vi "PM9_TCP_MODE.vi"(0 "VISA":refnum<visa-resource-name>="TCPIP0::169.254.70.190::502::SOCKET", 5 "connection ID":refnum<k5>, 11 "error in (no error)":errorcluster, 13 "MODE":u16(ring) items=["READ ONLY"=0, "AUTO"=10, "OFF"=62, "MAN"=54], 14 "Close tcp(t)":bool) -> (3 "mode(read)":string="OFF", 4 "visa out":refnum<visa-resource-name>, 6 "connection ID out":refnum<k5>, 15 "error out":errorcluster)   [LabVIEW 2018]
panel:
  # "Use a valid connection id to run in loop"
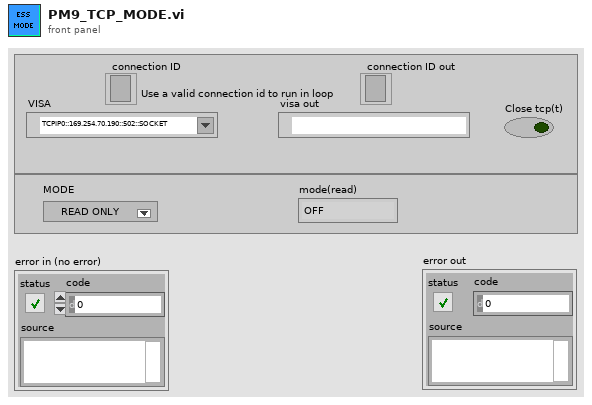
[diagram p1: front panel]
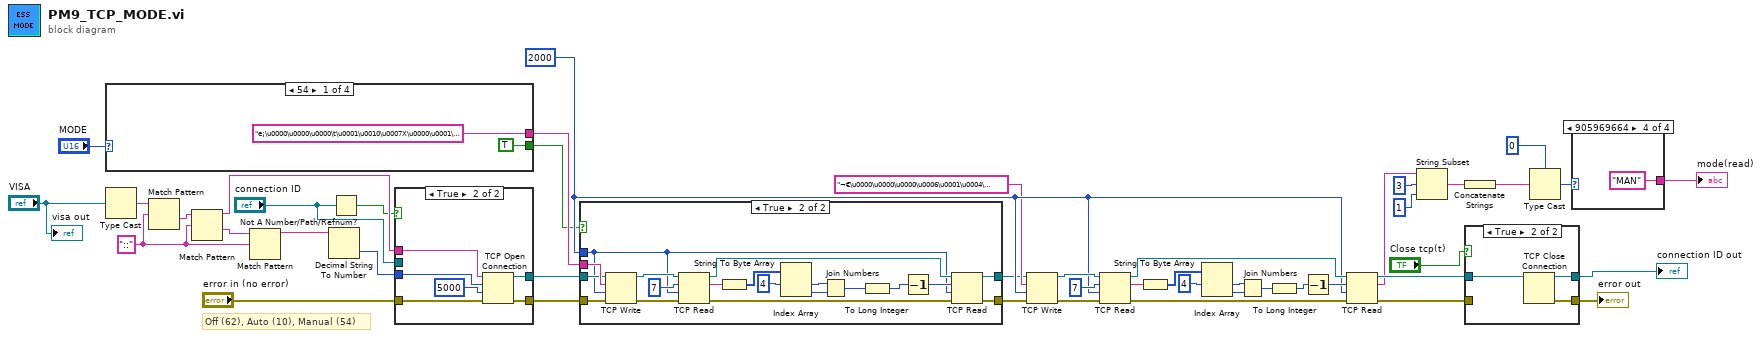
[diagram p0: block diagram]
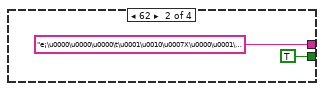
[diagram p3: hidden frame]
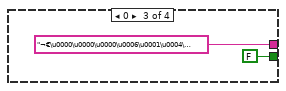
[diagram p4: hidden frame]
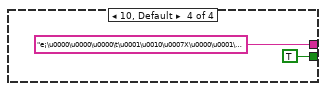
[diagram p5: hidden frame]
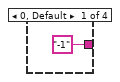
[diagram p6: hidden frame]
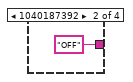
[diagram p7: hidden frame]
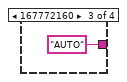
[diagram p8: hidden frame]
diagram:
  w38 = "::" ("search string/char (-)")
  w9 = 2000 ("timeout ms (25000)")
  # "Off (62), Auto (10), Manual (54)"
  n1 = case shown="54" "MODE" {
    tunnel: ["e¡\u0000\u0000\u0000\t\u0001\u0010\u0007X\u0000\u0001\u0002\u00006" ("address") "e¡\u0000\u0000\u0000\t\u0001\u0010\u0007X\u0000\u0001\u0002\u0000>" ("address") "¬€\u0000\u0000\u0000\u0006\u0001\u0004\u0007X\u0000\u0002" ("address") "e¡\u0000\u0000\u0000\t\u0001\u0010\u0007X\u0000\u0001\u0002\u0000\n" ("address")] -> w27
    tunnel: [TRUE TRUE FALSE TRUE] -> w5
    frame 54 {
    }
    frame 62 {
    }
    frame 0 {
    }
    frame 10, Default {
    }
  }
  n2 = Type Cast(x="VISA") -> (*(type *) &x=w41:string)  [unwired: 1 in]
  n3 = Match Pattern(string=w41, regular expression=w38) -> (after substring=w40:string)  [unwired: 1 in, 3 out]
  n4 = Match Pattern(string=w40, regular expression=w38) -> (before substring=w36:string, after substring=w39:string)  [unwired: 1 in, 2 out]
  n5 = Match Pattern(string=w39, regular expression=w38) -> (before substring=w37:string)  [unwired: 1 in, 3 out]
  n6 = Decimal String To Number(string=w37) -> (number=w35:i32)  [unwired: 2 in, 1 out]
  n7 = Not A Number/Path/Refnum?(number/path/refnum="connection ID") -> (NaN/Path/Refnum?=w30:bool)
  n8 = case shown="True" w30 {
    tunnel: [w56 w62] -> w4
    tunnel: [w55 w61] -> w46
    tunnel: w36 -> [_ w59]
    tunnel: w35 -> [_ w58]
    tunnel: "error in (no error)" -> [w55 w57]
    tunnel: "connection ID" -> [w56 _]
    frame False {
    }
    frame True {
      n9 = TCP Open Connection(address=w59, remote port or service name=w58, timeout ms (60000)=5000, error in (no error)=w57) -> (connection ID=w62:refnum<k5>, error out=w61:errorcluster)  [unwired: 1 in]
    }
  }
  n10 = case shown="True" w5 {
    tunnel: w46 -> [w64 w83]
    tunnel: w27 -> [_ w69]
    tunnel: w4 -> [w63 w68]
    tunnel: [w64 w67] -> w11
    tunnel: w9 -> [_ w66]
    tunnel: [w63 w65] -> w7
    frame False {
    }
    frame True {
      n11 = TCP Write(connection ID=w68, data in=w69, error in (no error)=w83, 9:w66) -> (connection ID out=w82:refnum<k5>, error out=w80:errorcluster)  [unwired: 1 out]
      n12 = TCP Read(connection ID=w82, bytes to read=7, error in (no error)=w80, 9:w66) -> (connection ID out=w81:refnum<k5>, data out=w71:string, error out=w79:errorcluster)  [unwired: 1 in]
      n13 = String To Byte Array(string=w71) -> (unsigned byte array=w72:u8[])
      n14 = Index Array(array=w72, index #1=4 ("index")) -> (element #1=w73:u8, element #2=w74:u8)  [unwired: 1 in]
      n15 = Join Numbers(hi=w73, lo=w74) -> ((hi.lo)=w76:u16)
      n16 = To Long Integer(number=w76) -> (32bit integer=w75:i32)
      n17 = Decrement(x=w75) -> (x-1=w70:i32)
      n18 = TCP Read(connection ID=w81, bytes to read=w70, error in (no error)=w79, 9:w66) -> (connection ID out=w65:refnum<k5>, error out=w67:errorcluster)  [unwired: 1 in, 1 out]
    }
  }
  n19 = TCP Write(connection ID=w7, data in="¬€\u0000\u0000\u0000\u0006\u0001\u0004\u0007X\u0000\u0002" ("address"), error in (no error)=w11, 9:w9) -> (connection ID out=w12:refnum<k5>, error out=w14:errorcluster)  [unwired: 1 out]
  n20 = TCP Read(connection ID=w12, bytes to read=7, error in (no error)=w14, 9:w9) -> (connection ID out=w13:refnum<k5>, data out=w23:string, error out=w15:errorcluster)  [unwired: 1 in]
  n21 = String To Byte Array(string=w23) -> (unsigned byte array=w22:u8[])
  n22 = Index Array(array=w22, index #1=4 ("index")) -> (element #1=w21:u8, element #2=w20:u8)  [unwired: 1 in]
  n23 = Join Numbers(hi=w21, lo=w20) -> ((hi.lo)=w18:u16)
  n24 = To Long Integer(number=w18) -> (32bit integer=w19:i32)
  n25 = Decrement(x=w19) -> (x-1=w24:i32)
  n26 = TCP Read(connection ID=w13, bytes to read=w24, error in (no error)=w15, 9:w9) -> (connection ID out=w6:refnum<k5>, data out=w3:string, error out=w10:errorcluster)  [unwired: 1 in]
  n27 = String Subset(string=w3, offset (0)=u16 3 ("offset"), length (rest)=u16 1 ("bytes to read")) -> (substring=w43:string)
  n28 = Concatenate Strings(w43) -> (w1:string)
  n29 = case shown="True" "Close tcp(t)" {
    tunnel: w6 -> [w85 w88]
    tunnel: [w84 w87] -> w25
    tunnel: [w85 w86] -> w33
    tunnel: w10 -> [w84 _]
    frame False {
    }
    frame True {
      n30 = TCP Close Connection(connection ID=w88) -> (connection ID out=w86:refnum<k5>, error out=w87:errorcluster)  [unwired: 2 in]
    }
  }
  "error out" <- w25
  "connection ID out" <- w33
  n31 = Type Cast(type=0, x=w1) -> (*(type *) &x=w29:i32)
  n32 = case shown="905969664" w29 {
    tunnel: ["-1" "OFF" "AUTO" "MAN"] -> w28
    frame 0, Default {
    }
    frame 1040187392 {
    }
    frame 167772160 {
    }
    frame 905969664 {
    }
  }
  "mode(read)" <- w28
  "visa out" <- "VISA"
